vi "Destroy.vi"(8 "error in (no error)":errorcluster, 11 "Driver":refnum<class "Driver.lvclass">) -> (0 "error out":errorcluster)   [LabVIEW 2020, in "Driver.lvclass"]
uses:
  Driver.lvclass
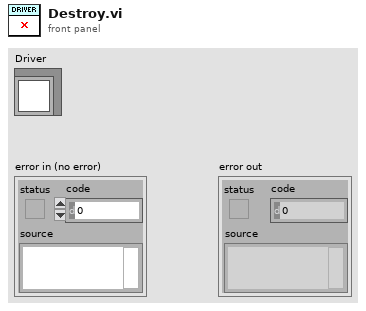
[diagram p1: front panel]
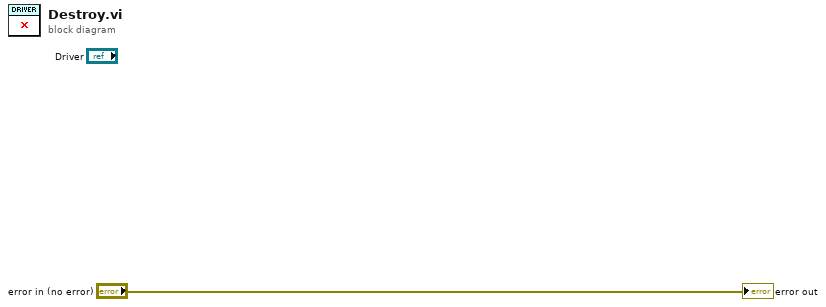
[diagram p0: block diagram]
diagram:
  "error out" <- "error in (no error)"
